vi "Read GainData.vi"(8 "error in (no error)":errorcluster, 11 "APDClass in":refnum<class "APDClass.lvclass">) -> (0 "error out":errorcluster, 2 "GainData":T1, 3 "APDClass out":refnum<class "APDClass.lvclass">)   [LabVIEW 2020, in "APDClass.lvclass"]
uses:
  APDClass.lvclass
  GainData.ctl
  APDClass.lvclass/APDClass.ctl
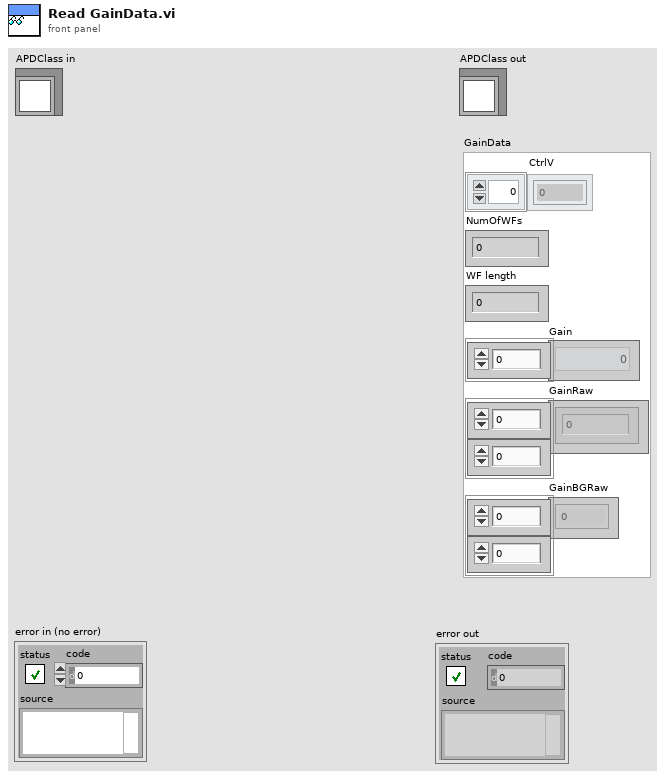
[diagram p1: front panel]
types:
  T1 = typedef "GainData.ctl" = cluster{"CtrlV":dbl[], "NumOfWFs":i32, "WF length":i32, "Gain":dbl[], "GainRaw":dbl[][], "GainBGRaw":dbl[][]}
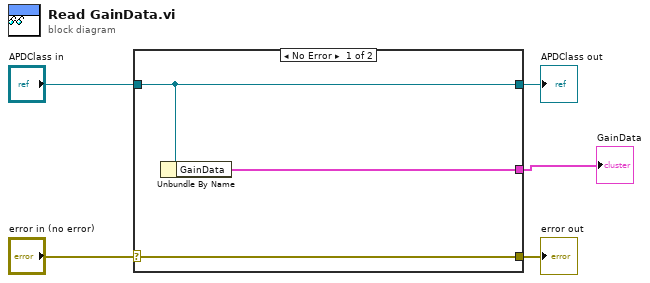
[diagram p0: block diagram]
diagram:
  n1 = case shown="No Error" "error in (no error)" {
    selector: "error in (no error)" -> [w8 w9]
    tunnel: [w8 w9] -> w4
    tunnel: [w7 w10] -> w2
    tunnel: "APDClass in" -> [w7 w10]
    tunnel: [w6 _] -> w1
    frame No Error {
      n2 = Unbundle By Name(w7) -> ("GainData"=w6:T1)
    }
    frame Error {
    }
  }
  "error out" <- w4
  "APDClass out" <- w2
  "GainData" <- w1
